vi "Open test manager.vi"(5 "enableDefaultFile":bool, 8 "error in (no error)":errorcluster, 11 "globalThreshold":T1=enum."INFO") -> (0 "error out":errorcluster, 3 "Logger out":refnum<class "Logger.lvclass">)   [LabVIEW 2026, in "Tests.lvlib"]
doc: "Launches a LogManager for integration tests with the default file appender disabled (enableDefaultFile FALSE), so the test controls exactly which appenders exist, then registers a RelayAppender in queue mode as a capture probe and returns the Logger instance plus the probe's queue. The test drives log calls through the Logger and dequeues delivered Statements from the queue to assert. Fixture, not a test."
uses:
  Tests.lvlib
  src/TypeDefs/Severity.ctl
  src/Public/Logger.lvclass/Logger.lvclass
  src/Lumberjack.lvlib
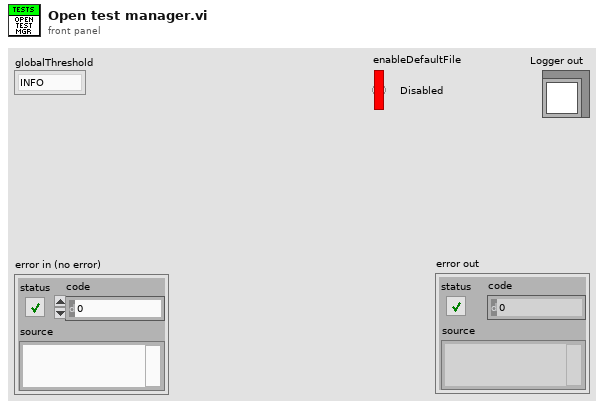
[diagram p1: front panel]
types:
  T1 = typedef "Lumberjack.lvlib/Severity.ctl" = enum16{"OFF", "FATAL", "ERROR", "WARN", "INFO", "DEBUG", "TRACE", "ALL"}
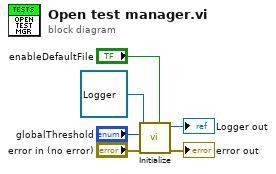
[diagram p0: block diagram]
diagram:
  n1 = call "Initialize.vi"("enableDefaultFile"="enableDefaultFile", "error in (no error)"="error in (no error)", "initialGlobalThreshold"="globalThreshold", "Logger in"=refnum<class "Logger.lvclass"> refnum) -> ("error out"=→"error out":errorcluster, "Logger out"=→"Logger out":refnum<class "Logger.lvclass">)  [unwired: 6 in]
